vi "SVFA Phase Unit Conversion (NxM).vi"(0 "phase spectra":cluster{"x0":dbl, "dx":dbl, "phase":dbl[]}[][](array[cluster]) {"phase" format="%.2p"; "dx" format="%.2p"; "x0" format="%.2p"}, 1 "desired units":T7(ring), 4 "spectrum info in":T1[][](array[typedef]) {"x-axis units" items=["Time (s)"=0, "Frequency-CB (Hz)"=1, "Frequency-CPB (Hz)"=1248, "Frequency-Arbitrary (Hz)"=2357, "Quefrency (s)"=2, "Revolutions (rev)"=3, "Order"=4, "Speed (RPM)"=11, "Speed (rad/s)"=21, "Index"=65535]; "weighting filter" items=["Linear", "A-weighting", "B-weighting", "C-weighting", "ITU-R 468-4", "Dolby", "CCITT", "C-message", "Wb", "Wc", "Wd", "We", "Wf", "Wh", "Wj", "Wk", "Wm", "AES17 20 kHz lowpass", "AES17 40 kHz lowpass", "AES17 20 kHz highpass", "AES17 40 kHz highpass"]; "dB reference [EU]" format="%.2f"; "engineering units" items=["custom..."=0, "V"=1, "A"=21, "C"=30, "pC"=31, "s"=32, "-"=29, "Pa"=2, "N"=20, "g"=3, "m/s^2"=4, "m/s"=5, "m"=6, "mm/s"=12, "mm"=13, "micron/s"=14, "micron"=15, "in/s^2"=7, "in/s"=8, "in"=9, "mil/s"=10, "mil"=11, "rad/s^2"=16, "rad/s"=17, "rad"=18, "deg/s^2"=26, "deg/s"=27, "deg"=28, "RPM"=22, "cycle/s^2"=23, "Hz"=24, "cycle"=25, "strain"=19]; "spectral info"."window" items=["None "=0, "Hanning"=1, "Hamming"=2, "Blackman-Harris"=3, "Exact Blackman"=4, "Blackman"=5, "Flat Top"=6, "4 Term B-Harris "=7, "7 Term B-Harris"=8, "Low Sidelobe"=9, "Force - Exponential"=10, "Gaussian"=62]}, 5 "error in (no error)":errorcluster) -> (14 "converted phase spectra":cluster{"x0":dbl, "dx":dbl, "phase":dbl[]}[][](array[cluster]) {"phase" format="%.2p"; "dx" format="%.2p"; "x0" format="%.2p"}, 15 "unit labels":string[][](array[string]), 18 "spectrum info out":T1[][](array[typedef]) {"x-axis units" items=["Time (s)"=0, "Frequency-CB (Hz)"=1, "Frequency-CPB (Hz)"=1248, "Frequency-Arbitrary (Hz)"=2357, "Quefrency (s)"=2, "Revolutions (rev)"=3, "Order"=4, "Speed (RPM)"=11, "Speed (rad/s)"=21, "Index"=65535]; "weighting filter" items=["Linear", "A-weighting", "B-weighting", "C-weighting", "ITU-R 468-4", "Dolby", "CCITT", "C-message", "Wb", "Wc", "Wd", "We", "Wf", "Wh", "Wj", "Wk", "Wm", "AES17 20 kHz lowpass", "AES17 40 kHz lowpass", "AES17 20 kHz highpass", "AES17 40 kHz highpass"]; "dB reference [EU]" format="%.2f"; "engineering units" items=["custom..."=0, "V"=1, "A"=21, "C"=30, "pC"=31, "s"=32, "-"=29, "Pa"=2, "N"=20, "g"=3, "m/s^2"=4, "m/s"=5, "m"=6, "mm/s"=12, "mm"=13, "micron/s"=14, "micron"=15, "in/s^2"=7, "in/s"=8, "in"=9, "mil/s"=10, "mil"=11, "rad/s^2"=16, "rad/s"=17, "rad"=18, "deg/s^2"=26, "deg/s"=27, "deg"=28, "RPM"=22, "cycle/s^2"=23, "Hz"=24, "cycle"=25, "strain"=19]; "spectral info"."window" items=["None "=0, "Hanning"=1, "Hamming"=2, "Blackman-Harris"=3, "Exact Blackman"=4, "Blackman"=5, "Flat Top"=6, "4 Term B-Harris "=7, "7 Term B-Harris"=8, "Low Sidelobe"=9, "Force - Exponential"=10, "Gaussian"=62]}, 19 "error out":errorcluster)   [LabVIEW 2017]
doc: "Converts phase spectra between degrees, radians, and cycles. Wire data to the <B>phase spectrum</B> input to determine the polymorphic instance to use or manually select the instance."
uses:
  <vilib>/addons/_NISVFA/_Shared subVIs/Controls/svc_Spectrum Info.ctl
  <vilib>/addons/_NISVFA/_Shared subVIs/Controls/svc_X-Axis Units.ctl
  <vilib>/addons/_NISVFA/_Shared subVIs/Controls/svc_Spectrum Type.ctl
  <vilib>/addons/_NISVFA/_Shared subVIs/Controls/svc_Engineering Units Text Ring.ctl
  <vilib>/addons/_NISVFA/_Shared subVIs/Controls/svc_Weighting Filter Text Ring.ctl
  <vilib>/addons/_NISVFA/_Shared subVIs/Controls/svc_Complimentary Spectrum Units.ctl
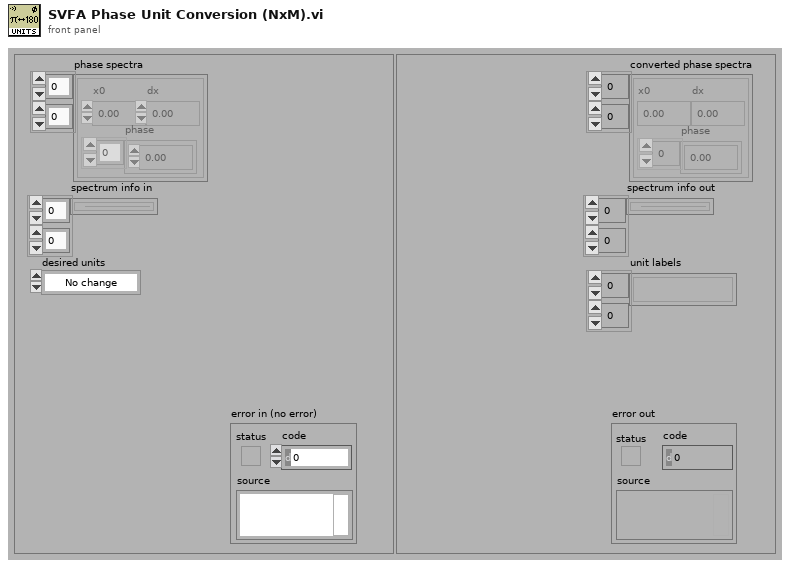
[diagram p1: front panel]
types:
  T1 = typedef "svc_Spectrum Info.ctl" = cluster{"channel name":string, "description":string, "x-axis units":T2, "spectral info":cluster{"spectrum type":T3, "linear/dB":enum16{"linear", "dB"}, "window":u16, "window size":i32, "FFT size":i32}, "engineering units":T4, "custom label":string, "dB reference [EU]":dbl, "peak units":enum16{"rms", "peak", "peak-peak"}, "weighting filter":T5, "spectral density?":bool, "unit label":string, "spectrum skewed?":bool, "complimentary spectrum units":T6}
  T2 = typedef "svc_X-Axis Units.ctl" = u16
  T3 = typedef "svc_Spectrum Type.ctl" = enum16{"FFT Spectrum [complex]", "Amplitude [Magnitude]", "Power [Magnitude^2]", "Cross Spectrum [complex]", "Frequency Response [Complex]"}
  T4 = typedef "svc_Engineering Units Text Ring.ctl" = u16
  T5 = typedef "svc_Weighting Filter Text Ring.ctl" = u16
  T6 = typedef "svc_Complimentary Spectrum Units.ctl" = enum16{"none", "radians", "degrees", "cycles", "imaginary"}
  T7 = enum16{"No change", "Radians", "Degrees", "Cycles"}
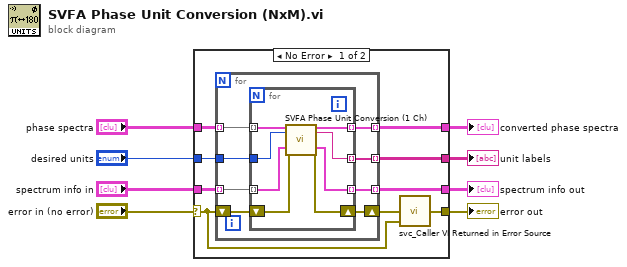
[diagram p0: block diagram]
diagram:
  n1 = case shown="No Error" "error in (no error)" {
    selector: "error in (no error)" -> [w9 w34]
    tunnel: "spectrum info in" -> [w17 w35]
    tunnel: "phase spectra" -> [w16 w36]
    tunnel: "desired units" -> [w15 _]
    tunnel: [w13 w34] -> w4
    tunnel: [w12 w35] -> w3
    tunnel: [w11 w36] -> w2
    tunnel: [w10 _] -> w1
    frame No Error {
      n2 = for {
        tunnel: w17 -> [w25] mode=indexing
        tunnel: w16 -> [w24] mode=indexing
        tunnel: w15 -> [w23]
        tunnel: [w21] -> w12 mode=indexing
        tunnel: [w20] -> w11 mode=indexing
        tunnel: [w19] -> w10 mode=indexing
        shift-right: [w22] -> w14
        shift-left: w9 -> [w18]
        n3 = for {
          tunnel: w25 -> [w33] mode=indexing
          shift-right: [w31] -> w22
          shift-left: w18 -> [w32]
          tunnel: w24 -> [w30] mode=indexing
          tunnel: w23 -> [w29]
          tunnel: [w28] -> w21 mode=indexing
          tunnel: [w27] -> w20 mode=indexing
          tunnel: [w26] -> w19 mode=indexing
          n4 = call <vilib>:"SVFA Phase Unit Conversion (1 Ch).vi"("phase spectrum"=w30, "desired units"=w29, "spectrum info in"=w33, "error in (no error)"=w32) -> ("converted phase spectrum"=w27:cluster{"f0":dbl, "df":dbl, "phase":dbl[]}, "unit label"=w26:string, "spectrum info out"=w28:T1, "error out"=w31:errorcluster)  [unwired: 12 in]
        }
      }
      n5 = call <vilib>:"svc_Caller VI Returned in Error Source.vi"("warning input to caller"=w9, "error in (no error)"=w14) -> ("error out"=w13:errorcluster)  [unwired: 3 in]
    }
    frame Error {
    }
  }
  "converted phase spectra" <- w2
  "error out" <- w4
  "spectrum info out" <- w3
  "unit labels" <- w1
